vi "CT-Test (interactive).vi"() -> ()   [LabVIEW 2015]
uses:
  CT-Params.ctl
  CT-Phase Enum.ctl
  <vilib>/sound2/lvsound2.llb/Sound Data Format.ctl
  <vilib>/sound2/lvsound2.llb/Sampling Mode.ctl
  <vilib>/Analysis/4window.llb/Hamming Window (DBL).vi
  <vilib>/Analysis/4window.llb/AllCosWindow (DBL).vi
  Utility VIs/Math VIs/FFT x(t) to dB,Degrees (1D).vi
  <vilib>/sound2/lvsound2.llb/Sound Output Write (DBL Single).vi
  <vilib>/Analysis/NI_AALPro.lvlib
panel:
  in  "stop":bool
  in  "F0 (Hz)":dbl(slide)=400.0 min=400.0 max=800.0 scale=400.0..800.0
  out "Time":cluster{"Array":dbl[], "Array":dbl[]}(graph)
  out "Freq":cluster{"Array":dbl[], "Array":dbl[]}(graph)
  in  "Frame size (ms)":dbl=50.0
  in  "Fs (Hz)":dbl=50000.0
  in  "HCT Params":T1={"F0 (Hz)"=500.0, "Band"={"Flow (Hz)"=800.0, "Fhigh (Hz)"=8000.0}, "Phase"=enum."Cosine", "Min F0 (Hz)"=400.0, "Max F0 (Hz)"=800.0, "ContinRandPhase"=FALSE, "Max peak factor"=inf, "Max mod depth"=2.0}
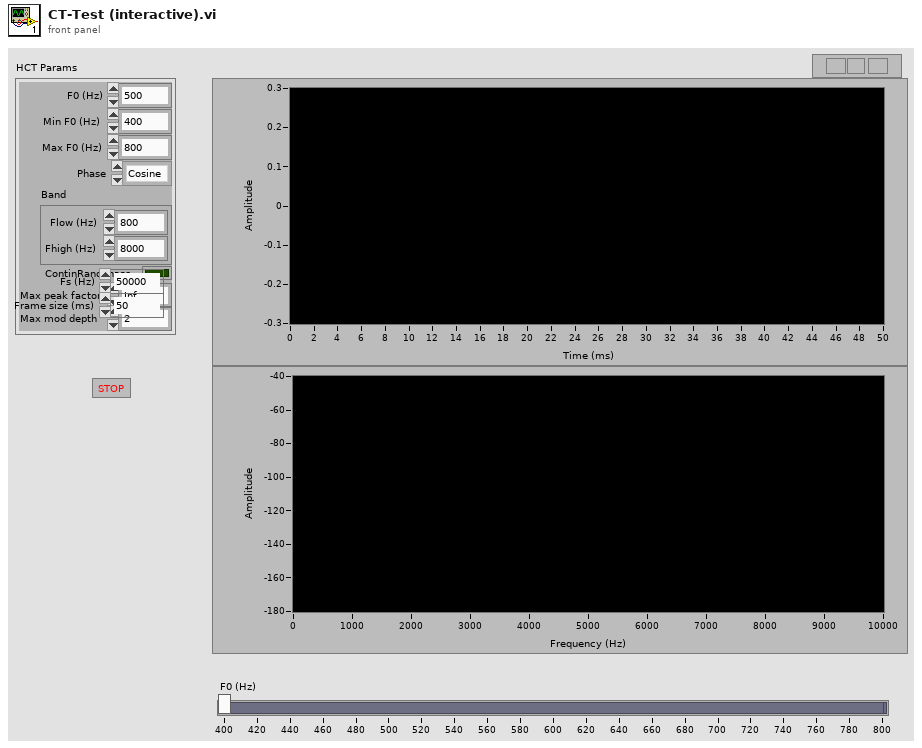
[diagram p1: front panel]
types:
  T1 = typedef "CT-Params.ctl" = cluster{"F0 (Hz)":dbl, "Band":cluster{"Flow (Hz)":dbl, "Fhigh (Hz)":dbl}, "Phase":T2, "Min F0 (Hz)":dbl, "Max F0 (Hz)":dbl, "ContinRandPhase":bool, "Max peak factor":dbl, "Max mod depth":dbl}
  T2 = typedef "CT-Phase Enum.ctl" = enum16{"Cosine", "Random", "Alternating"}
  T3 = typedef "Sampling Mode.ctl" = i32
  T4 = typedef "Sound Data Format.ctl" = cluster{"sample rate (S/s)":dbl, "number of channels":i32, "bits per sample":i32}
  T5 = typedef "CT-Runtime Data.ctl" = cluster{"Ncomp":i32, "MinHarm":i32, "Phase":dbl[], "Amplitude":dbl[], "Npts/frame":i32, "Last F0":dbl, "Fmin":dbl, "Fmax":dbl, "Lslope":dbl, "randphase":bool}
  T6 = typedef "Sound Output Task ID.ctl" = u32
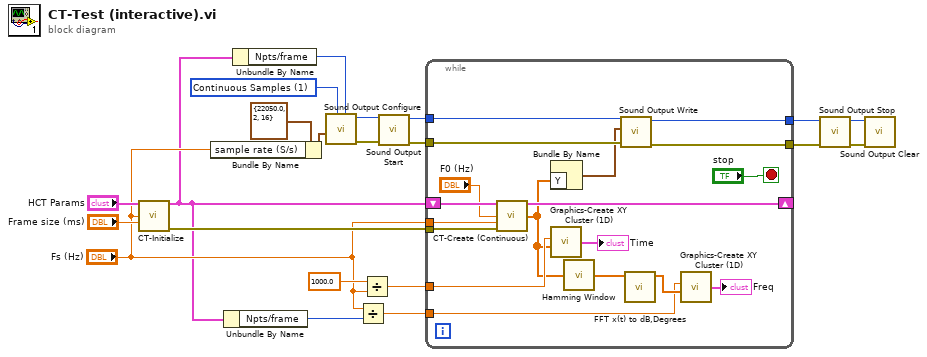
[diagram p0: block diagram]
diagram:
  w13 = T3 1 items=["Finite Samples", "Continuous Samples"] ("sample mode")
  n1 = call "CT-Initialize.vi"("HCT Params"="HCT Params", "Fs (Hz)"="Fs (Hz)", "Frame size (ms)"="Frame size (ms)") -> ("HCT Runtime"=w12:T5, "error out"=w20:errorcluster)  [unwired: 11 in]
  n2 = Bundle By Name(cluster=T4 {"sample rate (S/s)"=22050.0, "number of channels"=2, "bits per sample"=16} ("sound format"), "sample rate (S/s)"="Fs (Hz)") -> (w15:T4)
  n3 = Unbundle By Name(w12) -> ("Npts/frame"=w18:i32)
  n4 = Unbundle By Name(w12) -> ("Npts/frame"=w11:i32)
  n5 = call <vilib>:"Sound Output Configure.vi"("number of samples/ch"=w11, "sample mode"=w13, "sound format"=w15) -> ("error out"=w9:errorcluster, "task ID"=w10:T6)  [unwired: 7 in]
  n6 = Divide(x="Fs (Hz)", y=w18) -> (x/y=w1:dbl)
  n7 = Divide(x=1000.0, y="Fs (Hz)") -> (x/y=w2:dbl)
  n8 = call <vilib>:"Sound Output Start.vi"("error in (no error)"=w9, "task ID"=w10) -> ("error out"=w7:errorcluster, "task ID out"=w8:T6)  [unwired: 8 in]
  n9 = while {
    tunnel: w20 -> [w39]
    tunnel: "Fs (Hz)" -> [w38]
    shift-right: [w36] -> _
    shift-left: w12 -> [w37]
    tunnel: w8 -> [w32]
    tunnel: w7 -> [w31]
    tunnel: [w29] -> w6
    tunnel: [w28] -> w5
    tunnel: w2 -> [w27]
    tunnel: w1 -> [w23]
    stop <- "stop" stop-if-true
    n10 = call "CT-Create (Continuous).vi"("HCT Runtime in"=w37, "F0 (Hz)"="F0 (Hz)", "Fs (Hz)"=w38, "error in (no error)"=w39) -> ("HCT Runtime out"=w36:T5, "HCT"=w26:dbl[])  [unwired: 9 in, 1 out]
    n11 = Bundle By Name("Y"=w26) -> (w30:waveform(dbl))  [unwired: 1 in]
    n12 = call "Graphics-Create XY Cluster (1D).vi"("Array"=w26, "dx"=w27) -> ("XY cluster"=→"Time":cluster{"Array":dbl[], "Array":dbl[]})  [unwired: 2 in]
    n13 = call-poly <vilib>:"Hamming Window.vi"("X"=w26) -> ("Windowed X"=w22:dbl[])  [unwired: 1 out]
    n14 = call-poly <vilib>:"Sound Output Write.vi"("error in (no error)"=w31, "data"=w30, "task ID"=w32) -> ("error out"=w28:errorcluster, "task ID out"=w29:T6)  [unwired: 7 in]
    n15 = call-poly "FFT x(t) to dB,Degrees.vi"("X"=w22) -> ("+Freq. Mag of FFT (dB rms)"=w24:dbl[])  [unwired: 8 in, 2 out]
    n16 = call "Graphics-Create XY Cluster (1D).vi"("Array"=w24, "dx"=w23) -> ("XY cluster"=→"Freq":cluster{"Array":dbl[], "Array":dbl[]})  [unwired: 2 in]
  }
  n17 = call <vilib>:"Sound Output Stop.vi"("error in (no error)"=w5, "task ID"=w6) -> ("error out"=w4:errorcluster, "task ID out"=w3:T6)  [unwired: 8 in]
  n18 = call <vilib>:"Sound Output Clear.vi"("error in (no error)"=w4, "task ID"=w3) -> ()  [unwired: 9 in, 1 out]
